vi "gfitsio-close-file.vi"(8 "error in (no error)":errorcluster, 11 "gfits refnum":T1) -> (0 "error out":errorcluster, 3 "Path":path)   [LabVIEW 2014, in "gfitsio.lvlib"]
doc: "Closes an open file specified by <B>gfits refnum</B>. Error I/O operates uniquely in this function, which closes the file regardless of whether an error occurred in a preceding operation."
uses:
  gfitsio/gfitsio.lvlib
  gfitsio-refnum.ctl
  gfitsio/gfitsio.dll
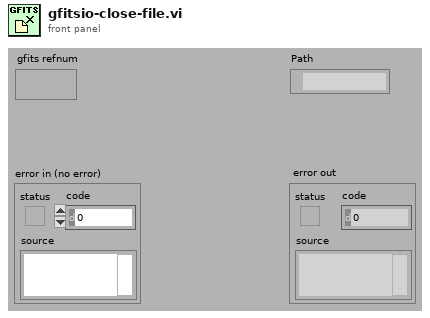
[diagram p1: front panel]
types:
  T1 = typedef "gfitsio.lvlib/gfitsio-refnum.ctl" = refnum<k1>
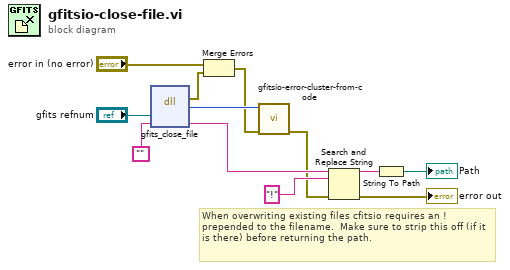
[diagram p0: block diagram]
diagram:
  # "When overwriting existing files cfitsio requires an ! prepended to the filename.  Make sure to strip this off (if it is there) before returning the path."
  n1 = dll-call lib="F:/labview_codes/labview_codes/gfitsio/gfitsio.dll" fn="gfits_close_file"("gfits refnum"="gfits refnum", "path"="") -> (error out=w4:errorcluster, w12:i32, "path"=w7:string)  [unwired: 4 in, 1 out]
  n2 = Merge Errors("error in (no error)", w4) -> (w3:errorcluster)
  n3 = call "gfitsio-error-cluster-from-code.vi"("error in (no error)"=w3, "error code"=w12) -> ("error out"=w2:errorcluster)  [unwired: 9 out]
  n4 = Search and Replace String(input string=w7, search string="!", error in=w2) -> (result string=w6:string, error out=→"error out":errorcluster)  [unwired: 5 in, 2 out]
  n5 = String To Path(string=w6) -> (path=→"Path":path)
